vi "Build State String with Arguments.vi"(4 "Arguments (\"\")":string, 5 "State":string) -> (1 "State with Arguments":string)   [LabVIEW 2013, in "JKI State Machine.lvlib"]
doc: "Builds a state string that contains arguments for the JKI State Machine.\n<B>For Example:</B> If State = A and Arguments = B then State with Arguments = A >> B\n\nFor instructions on how to use the JKI State Machine, examples and video tutorials, visit:\nhttp://jkisoft.com/state-machine/\n\n<B>Inputs:</B>\n <B>State:</B> The State string that requires the argument.\n <B>Arguments:</B> The Argument string to add to the state. The default is an empty string. If Argument is an empty string then State will be returned to the output. <B>Note:</B> The arguments input must not contain any unprintable characters like linefeed or carriage return.\n\n<B>Outputs:</B>\n <B>State with Arguments:</B> This output returns the new string that contains the State and the Argument. <B>For Example:</B> If State = A and Arguments = B then State with Arguments = A >> B\n\nJKI State Machine™\nhttp://jkisoft.com/state-machine/\nCopyright (C) 2005-2008, JKI <info@jkisoft.com>\nALL RIGHTS RESERVED"
uses:
  JKI State Machine.lvlib
panel:
  # "For instructions on how to use the JKI State Machine, examples and video tutorials, visit:\nhttp://jkisoft.com/state-machine/\n\nJKI State Machine™\nhttp://jkisoft.com/state-machine/\nCopyright (C) 2005-2008, JKI <info@jkisoft.com>\nALL RIGHTS RESERVED"
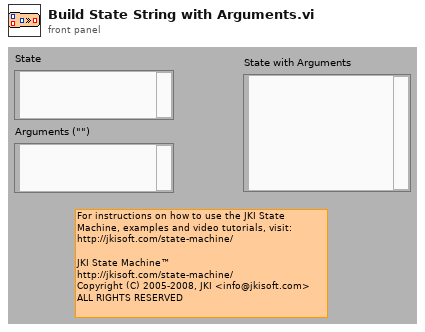
[diagram p1: front panel]
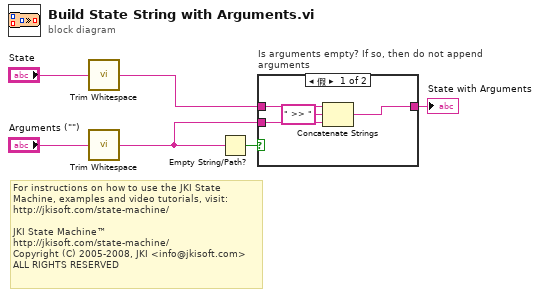
[diagram p0: block diagram]
diagram:
  # "For instructions on how to use the JKI State Machine, examples and video tutorials, visit:\nhttp://jkisoft.com/state-machine/\n\nJKI State Machine™\nhttp://jkisoft.com/state-machine/\nCopyright (C) 2005-2008, JKI <info@jkisoft.com>\nALL RIGHTS RESERVED"
  n1 = call <vilib>:"Trim Whitespace.vi"("string"="State") -> ("trimmed string"=w3:string)  [unwired: 1 in]
  n2 = call <vilib>:"Trim Whitespace.vi"("string"="Arguments (\"\")") -> ("trimmed string"=w2:string)  [unwired: 1 in]
  n3 = Empty String/Path?(string/path=w2) -> (empty?=w1:bool)
  n4 = case "Is arguments empty? If so, then do not append arguments" shown="假" w1 {
    tunnel: [w7 w11] -> w4
    tunnel: w3 -> [w10 w11]
    tunnel: w2 -> [w8 _]
    frame False {
      n5 = Concatenate Strings(w10, " >> " ("string"), w8) -> (w7:string)
    }
    frame True {
    }
  }
  "State with Arguments" <- w4
